vi "Free Memory.vi"(4 "error in (no error)":errorcluster, 7 "Pointer":i32) -> (0 "error out":errorcluster)   [LabVIEW 2011]
doc: "Use this VI to explicitely free memory allocated using the <B>Allocate Memory.VI</B>. Memory which is not freed using this VI will not be freed by the Operating System until the LabVIEW application is terminated."
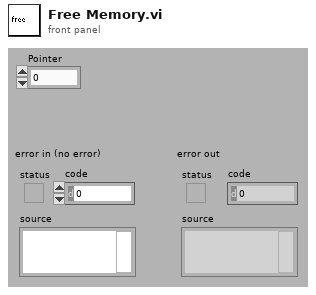
[diagram p1: front panel]
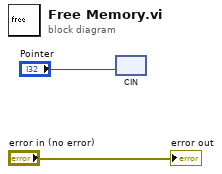
[diagram p0: block diagram]
diagram:
  n1 = cin("Pointer") -> ()  [unwired: 1 in]
  "error out" <- "error in (no error)"
